vi "3.4.2.vi"() -> ()   [LabVIEW 2018]
panel:
  out "최대 인덱스":i32
  out "최소값":dbl
  out "최소 인덱스":i32
  out "최대값":dbl
  out "뒤집힌 배열":dbl[](array[numeric])
  out "두 번째 부분배열":dbl[](array[numeric])
  out "첫 번째 부분배열":dbl[](array[numeric])
  out "정렬된 배열":dbl[](array[numeric])
  in  "배열":dbl[](array[numeric])
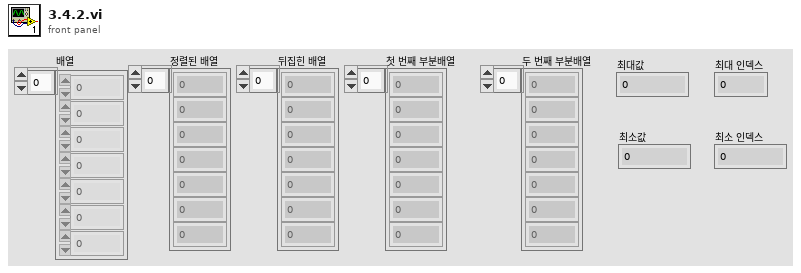
[diagram p1: front panel]
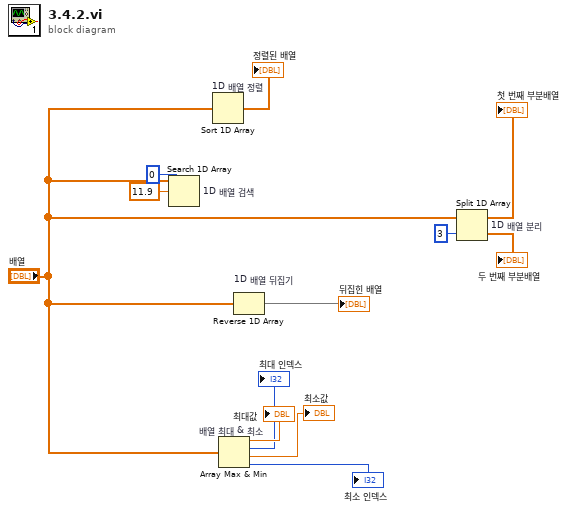
[diagram p0: block diagram]
diagram:
  n1 = Search 1D Array "1D 배열 검색"(1D array="배열", element=11.9 ("원소"), start index (0)=0 ("시작 인덱스(0)")) -> ()  [unwired: 1 out]
  n2 = Sort 1D Array "1D 배열 정렬"(array="배열") -> (sorted array=→"정렬된 배열":dbl[])
  n3 = Array Max & Min "배열 최대 & 최소"(array="배열") -> (max value=→"최대값":dbl, max index (indices)=→"최대 인덱스":i32, min value=→"최소값":dbl, min index (indices)=→"최소 인덱스":i32)
  n4 = Reverse 1D Array "1D 배열 뒤집기"(array="배열") -> (reversed array=→"뒤집힌 배열":dbl[])
  n5 = Split 1D Array "1D 배열 분리"(array="배열", index=3 ("인덱스")) -> (first subarray=→"첫 번째 부분배열":dbl[], second subarray=→"두 번째 부분배열":dbl[])
